vi "Configure Lamp Energy.vi"(7 "lamp (primary)":u16(ring)=1 items=["primary"=1, "secondary"=2], 8 "error in (no error)":errorcluster, 10 "energy, J":dbl, 11 "Lotis in":refnum<class "PL Lotis TII LS.lvclass">) -> (0 "error out":errorcluster, 3 "Lotis out":refnum<class "PL Lotis TII LS.lvclass">)   [LabVIEW 2015, in "PL Lotis TII LS.lvclass"]
doc: "Configures lamp energy."
uses:
  PL Lotis TII LS.lvclass
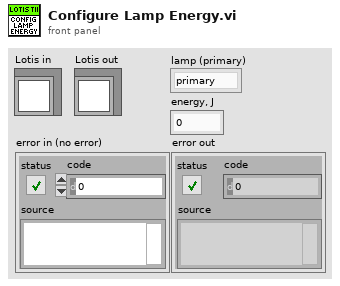
[diagram p1: front panel]
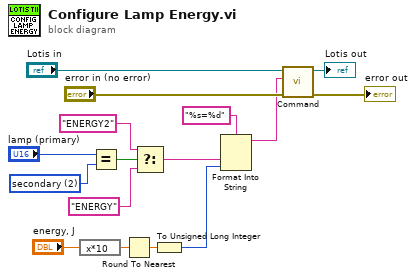
[diagram p0: block diagram]
diagram:
  w8 = u16 2 items=["primary"=1, "secondary"=2] ("lamp (primary) 2")
  n1 = expression code="x*10"("energy, J") -> (w3:dbl)
  n2 = Equal?(x="lamp (primary)", y=w8) -> (x = y?=w7:bool)
  n3 = Round To Nearest(number=w3) -> (nearest integer value=w2:dbl)
  n4 = Select(t="ENERGY2" ("input 1"), s=w7, f="ENERGY" ("input 1")) -> (s? t:f=w4:string)
  n5 = To Unsigned Long Integer(number=w2) -> (unsigned 32bit integer=w1:u32)
  n6 = Format Into String(format string="%s=%d" ("command"), w4, w1) -> (resulting string=w11:string)  [unwired: 2 in, 1 out]
  n7 = call "Command.vi"("error in (no error)"="error in (no error)", "command"=w11, "Lotis in"="Lotis in") -> ("error out"=→"error out":errorcluster, "Lotis out"=→"Lotis out":refnum<class "PL Lotis TII LS.lvclass">)  [unwired: 6 in, 1 out]
